vi "sort.volumes.vi"(11 "volumes":T1[](array[typedef])) -> (1 "end date":timestamp, 2 "start date":timestamp, 3 "volumes by row":cluster{"Array":T1[]}[](array[cluster]))   [LabVIEW 2024]
uses:
  CV_Shared_Library/volume.object--cluster.ctl
  CV_Shared_Library/volume.type--enum.ctl
  comic_manager/TypeDefs/issue.display--cluster.ctl
  CV_Shared_Library/CV_Shared_Library.lvlib
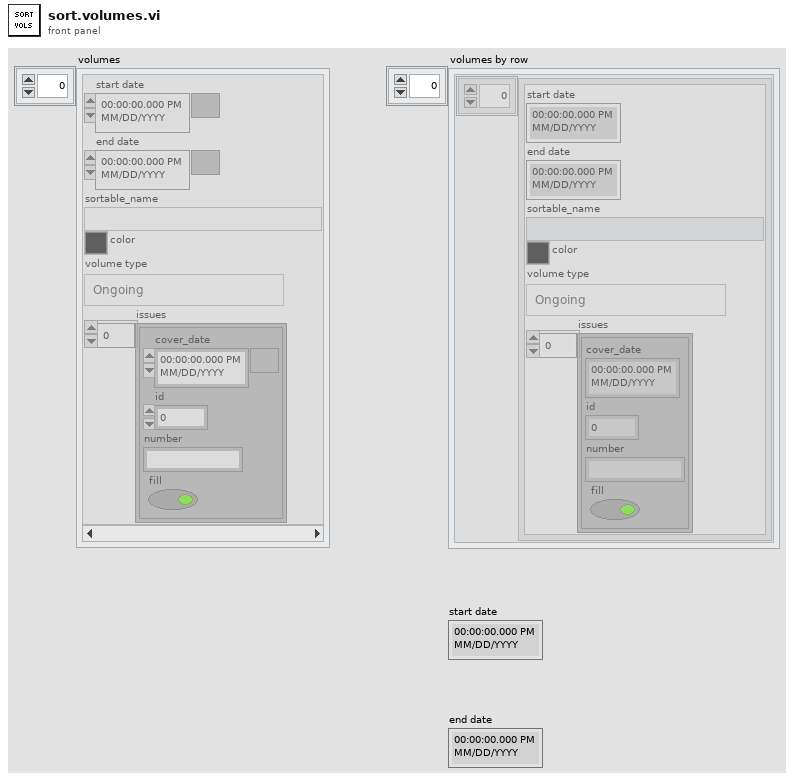
[diagram p1: front panel]
types:
  T1 = typedef "CV_Shared_Library.lvlib/volume.object--cluster.ctl" = cluster{"start date":timestamp, "end date":timestamp, "sortable_name":string, "color":u32, "volume type":T2, "issues":T3[]}
  T2 = typedef "CV_Shared_Library.lvlib/volume.type--enum.ctl" = enum16{"Ongoing", "Limited Series", "Annual", "One Shot", "Reprint/Document", "Star Comics", "Epic Comics"}
  T3 = typedef "CV_Shared_Library.lvlib/issue.display--cluster.ctl" = cluster{"cover_date":timestamp, "id":i32, "number":string, "fill":bool}
  T4 = cluster{"appended array":T1[], cluster{"open start":timestamp, "open end":timestamp}[]}[]
  T5 = cluster{"open start":timestamp, "open end":timestamp}
  T6 = cluster{"open start":timestamp, "open end":timestamp}[]
  T7 = cluster{"appended array":T1[], cluster{"open start":timestamp, "open end":timestamp}[]}
  T8 = cluster{T1[], cluster{"open start":timestamp, "open end":timestamp}[]}
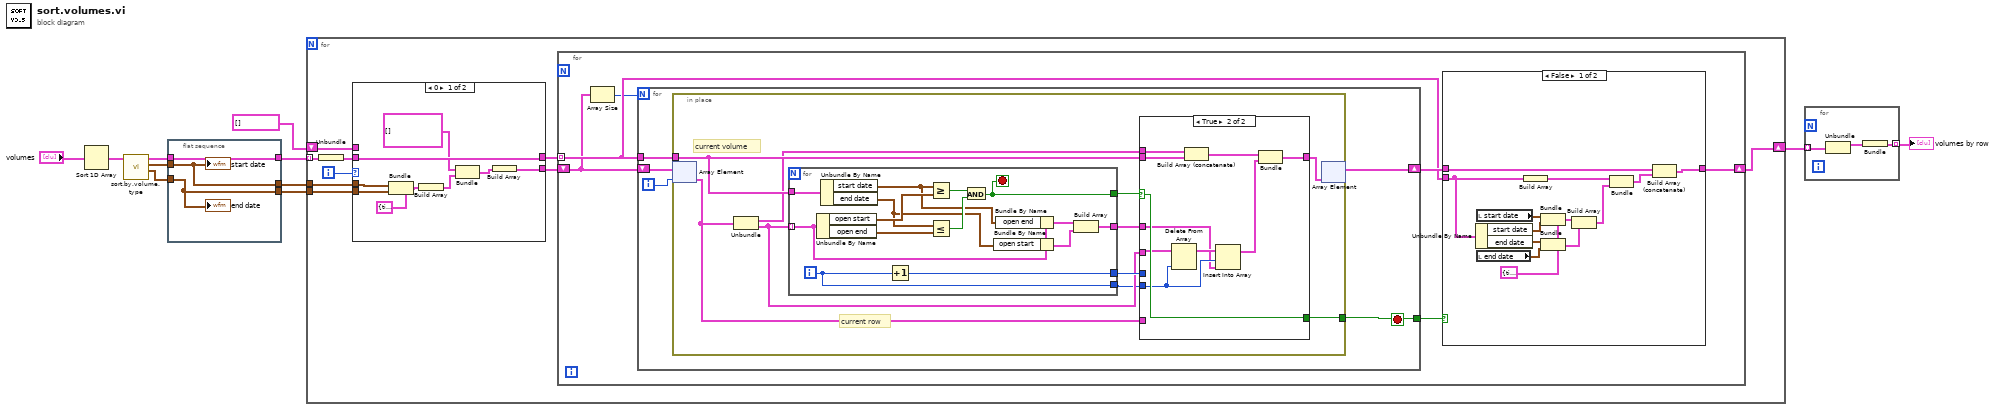
[diagram p0: block diagram]
diagram:
  n1 = Sort 1D Array(array="volumes") -> (sorted array=w10:T1[])
  n2 = call "sort.by.volume.type.vi"("Array in"=w10) -> ("end date"=w4:timestamp, "start date"=w5:timestamp, "Array"=w7:cluster{T1[]}[])  [unwired: 8 in]
  n3 = flat-sequence {
    tunnel: w7 -> [w14]
    tunnel: [w14] -> w6
    tunnel: w5 -> [w12]
    tunnel: w4 -> [w13]
    tunnel: [w13] -> w3
    tunnel: [w12] -> w2
    frame #0 {
      "start date" <- w12
      "end date" <- w13
    }
  }
  n4 = for {
    tunnel: w6 -> [w21] mode=indexing
    shift-right: [w19] -> w9
    shift-left: T4 [] -> [w17]
    tunnel: w3 -> [w16]
    tunnel: w2 -> [w15]
    i -> [w18]
    n5 = Unbundle(w21) -> (w20:T1[])
    n6 = case shown="0" w18 {
      tunnel: [w30 w33] -> w23
      tunnel: [w31 w34] -> w22
      tunnel: w20 -> [w30 w33]
      tunnel: w17 -> [_ w34]
      tunnel: w16 -> [w25 _]
      tunnel: w15 -> [w24 _]
      frame 0 {
        n7 = Bundle(cluster=T5 {"open start"=timestamp(0 s since 1904-01-01), "open end"=timestamp(0 s since 1904-01-01)}, "open start"=w24, "open end"=w25) -> (w28:T5)
        n8 = Build Array(w28) -> (w29:T6)
        n9 = Bundle("appended array"=T1[] [], w29) -> (w32:T7)  [unwired: 1 in]
        n10 = Build Array(w32) -> (w31:T4)
      }
      frame Default {
      }
    }
    n11 = for {
      tunnel: w23 -> [w37] mode=indexing
      shift-right: [w38] -> w19
      shift-left: w22 -> [w36]
      n12 = Array Size(array=w36) -> (size(s)=w35:i32)
      n13 = for {
        N: w35 -> [_]
        tunnel: w37 -> [w59]
        shift-right: [w57] -> w39
        shift-left: w36 -> [w58]
        tunnel: [w56] -> w40
        i -> [w55]
        stop <- w56 stop-if-true
        n14 = in-place {
          in-place-border: [w69] -> w56
          in-place-border: w59 -> [w66]
          # "current row"
          # "current volume"
          n15 = in-place-array #1(w58, w55) -> (w67:T7)
          n16 = Unbundle(w67) -> ("appended array"=w64:T1[], w62:T6)
          n17 = for {
            tunnel: w66 -> [w83]
            tunnel: [w79] -> w65
            tunnel: [w72] -> w63
            tunnel: w62 -> [w77] mode=indexing
            tunnel: [w76] -> w60
            tunnel: [w75] -> w61
            i -> [w75]
            stop <- w79 stop-if-true
            n18 = Unbundle By Name(w77) -> ("open start"=w78:timestamp, "open end"=w82:timestamp)
            n19 = Unbundle By Name(w83) -> ("start date"=w71:timestamp, "end date"=w70:timestamp)
            n20 = Increment(x=w75) -> (x+1=w72:i32)
            n21 = Greater Or Equal?(x=w71, y=w78) -> (x >= y?=w81:bool)
            n22 = Less Or Equal?(x=w70, y=w82) -> (x <= y?=w80:bool)
            n23 = And(x=w81, y=w80) -> (x .and. y?=w79:bool)
            n24 = Bundle By Name(cluster=w77, "open start"=w70) -> (w73:T5)
            n25 = Bundle By Name(cluster=w77, "open end"=w71) -> (w74:T5)
            n26 = Build Array(w74, w73) -> (w76:T6)
          }
          n27 = case shown="True" w65 {
            selector: w65 -> [w84 w95]
            tunnel: [w84 w95] -> w69
            tunnel: w64 -> [_ w93]
            tunnel: w66 -> [_ w92]
            tunnel: [w85 w94] -> w68
            tunnel: w67 -> [w85 _]
            tunnel: w63 -> [_ _]
            tunnel: w62 -> [_ w90]
            tunnel: w61 -> [_ w88]
            tunnel: w60 -> [_ w87]
            frame False {
            }
            frame True {
              n28 = Delete From Array(array=w90, index=w88) -> (array with subset deleted=w89:T6)  [unwired: 1 in, 1 out]
              n29 = Build Array (concatenate)(w93, w92) -> (w91:T1[])
              n30 = Insert Into Array(array=w89, index=w88, new element=w87) -> (w86:T6)
              n31 = Bundle(w91, w86) -> (w94:T8)  [unwired: 1 in]
            }
          }
          n32 = in-place-array #1(w68) -> (w57:T4)  [unwired: 1 out]
        }
      }
      n33 = case shown="False" w40 {
        tunnel: [w52 w54] -> w38
        tunnel: w39 -> [w53 w54]
        tunnel: w37 -> [w47 _]
        frame False {
          w44 = T5 {"open start"=timestamp(0 s since 1904-01-01), "open end"=timestamp(0 s since 1904-01-01)}
          n34 = Unbundle By Name(w47) -> ("start date"=w46:timestamp, "end date"=w43:timestamp)
          n35 = local read "start date"() -> (w48:timestamp)
          n36 = local read "end date"() -> (w41:timestamp)
          n37 = Build Array(w47) -> (w51:T1[])
          n38 = Bundle(cluster=w44, "open start"=w48, "open end"=w46) -> (w45:T5)
          n39 = Bundle(cluster=w44, "open start"=w43, "open end"=w41) -> (w42:T5)
          n40 = Build Array(w45, w42) -> (w50:T6)
          n41 = Bundle(w51, w50) -> (w49:T8)  [unwired: 1 in]
          n42 = Build Array (concatenate)(w53, w49) -> (w52:T4)
        }
        frame True {
        }
      }
    }
  }
  n43 = for {
    tunnel: w9 -> [w98] mode=indexing
    tunnel: [w96] -> w8 mode=indexing
    n44 = Unbundle(w98) -> ("appended array"=w97:T1[])  [unwired: 1 out]
    n45 = Bundle("appended array"=w97) -> (w96:cluster{"appended array":T1[]})  [unwired: 1 in]
  }
  "volumes by row" <- w8
